vi "DHMS - Converter.vi"() -> ()   [LabVIEW 2023]
panel:
  in  "?":bool
  out "Seconds":dbl
  out "Minutes":dbl
  out "Hours":dbl
  out "Days":dbl
  in  "Time s":dbl format="%#_6f"
  out "%Days":dbl format="%.2f"
  out "%Hours":dbl
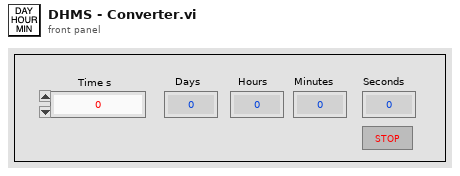
[diagram p1: front panel]
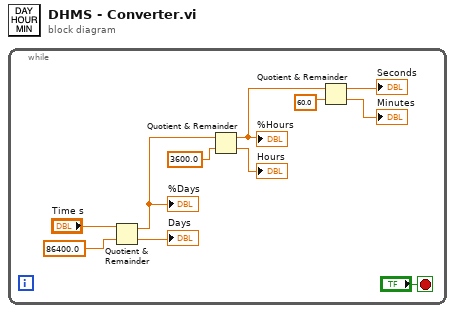
[diagram p0: block diagram]
diagram:
  n1 = while {
    stop <- "?" stop-if-true
    n2 = Quotient & Remainder(x="Time s", y=86400.0) -> (x-y*floor(x/y)=w8:dbl, floor(x/y)=→"Days":dbl)
    "%Days" <- w8
    n3 = Quotient & Remainder(x=w8, y=3600.0) -> (x-y*floor(x/y)=w5:dbl, floor(x/y)=→"Hours":dbl)
    "%Hours" <- w5
    n4 = Quotient & Remainder(x=w5, y=60.0) -> (x-y*floor(x/y)=→"Seconds":dbl, floor(x/y)=→"Minutes":dbl)
  }
